vi "AnalyseHeadImpulse2.vi"(0 "head velocity":dbl[](graph), 1 "impulse analysis params":T2={"No. baseline pts"=100, "threshhold"=10.0, "segment length"=300} {"threshhold" format="%.2f"}, 2 "Impulse Analysis Params":T1={"unfiltered vel?"=FALSE, "remove offset? (T)"=FALSE, "analysis method"=enum."polynomial fit", "pre-impulse position"=50, "post-impulse position"=50, "HIT axis"=enum."Pitch", "pre-impulse pts"=50, "post-impulse pts"=50, "polynomial order"=15, "algorithm"=enum."Givens"}, 5 "eye velocity":dbl[](graph), 11 "error in (no error)":errorcluster) -> (3 "impulse analysis params copy":T2={"No. baseline pts"=100, "threshhold"=10.0, "segment length"=9} {"threshhold" format="%.2f"}, 4 "extracted head impulse":dbl[](graph), 6 "extracted eye response":dbl[](graph), 14 "impulse analysis results":T3={"baseline intercept"=3.0, "impulse peak X"=352.0, "len"=400, "+ve ?"=TRUE, "peak velocity"=235.7274415929559} {"peak velocity" format="%.2f"; "impulse peak X" format="%.2f"; "baseline intercept" format="%.2f"}, 15 "error out":errorcluster)   [LabVIEW 2014, in "impulse functions.lvlib"]
uses:
  impulse functions.lvlib
  <vilib>/Analysis/1siggen.llb/Ramp Pattern by Samples.vi
  <vilib>/Analysis/NI_AALPro.lvlib
  <vilib>/Analysis/NI_AALBase.lvlib
panel:
  out "fit segment":dbl[][](graph)
  out "error":i32
  out "mse":dbl format="%.2f"
  out "Polynomial Fit Coefficients":dbl[](array[numeric]) format="%.2f"
  # "Copyright Americo A. Migliaccio (c) 2002 All Rights Reserved by Author"
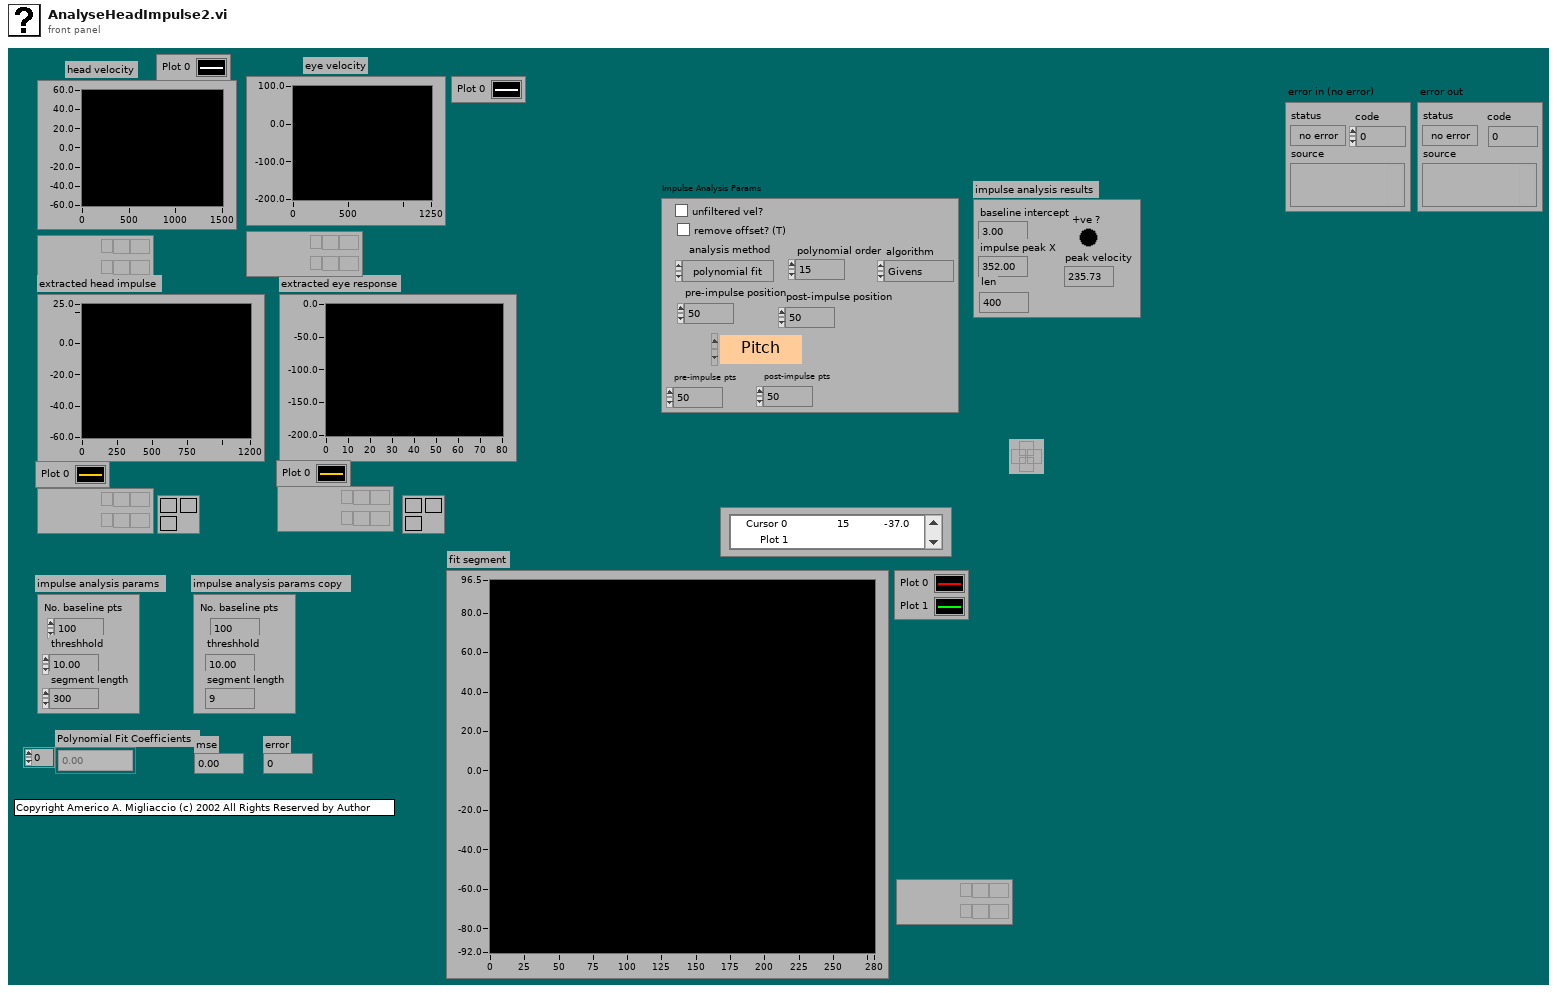
[diagram p1: front panel]
types:
  T1 = cluster{"unfiltered vel?":bool, "remove offset? (T)":bool, "analysis method":enum16{"original", "polynomial fit"}, "pre-impulse position":i32, "post-impulse position":i32, "HIT axis":enum16{"Yaw", "Pitch", "Roll"}, "pre-impulse pts":i32, "post-impulse pts":i32, "polynomial order":i32, "algorithm":enum32{"SVD", "Givens", "Givens2", "Householder", "LU Decomposition", "Cholesky"}}
  T2 = cluster{"No. baseline pts":i32, "threshhold":dbl, "segment length":i32}
  T3 = cluster{"baseline intercept":dbl, "impulse peak X":dbl, "len":i32, "+ve ?":bool, "peak velocity":dbl}
  T4 = enum32{"SVD", "Givens", "Givens2", "Householder", "LU Decomposition", "Cholesky"}
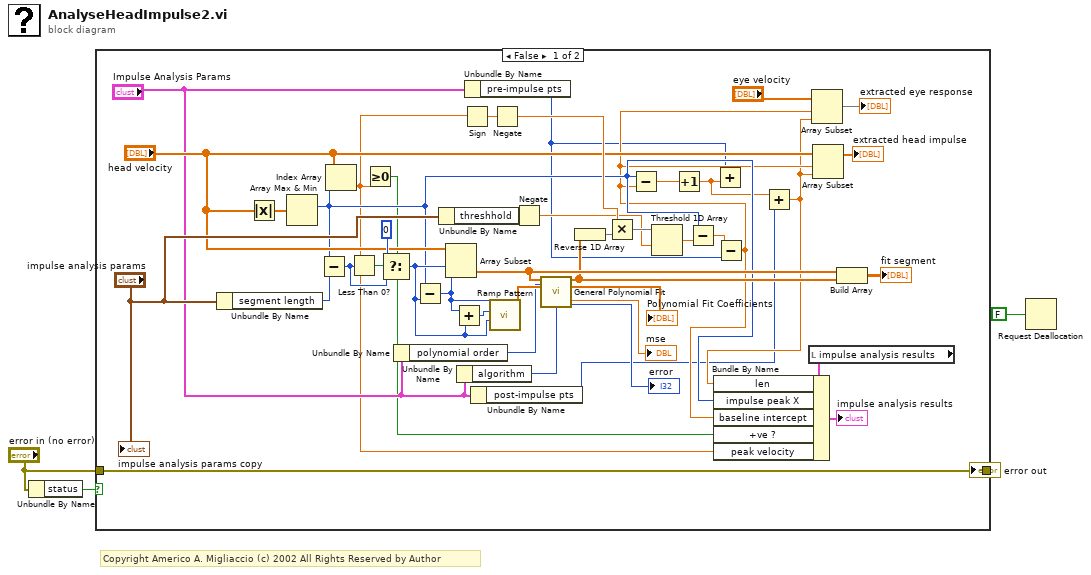
[diagram p0: block diagram]
diagram:
  # "Copyright Americo A. Migliaccio (c) 2002 All Rights Reserved by Author"
  n1 = Unbundle By Name("error in (no error)") -> ("status"=w4:bool)
  n2 = case shown="False" w4 {
    tunnel: "error in (no error)" -> [w40 w48]
    tunnel: [w40 w48] -> w2
    frame False {
      n3 = Unbundle By Name("impulse analysis params") -> ("segment length"=w33:i32)
      n4 = Absolute Value(x="head velocity") -> (abs(x)=w45:dbl[])
      n5 = Array Max & Min(array=w45) -> (max index (indices)=w17:i32)  [unwired: 3 out]
      n6 = Subtract(x=w17, y=w33) -> (x-y=w30:i32)
      n7 = Index Array(array="head velocity", index=w17) -> (element=w5:dbl)
      n8 = Less Than 0?(x=w30) -> (x < 0?=w32:bool)
      n9 = Greater Or Equal To 0?(x=w5) -> (x >= 0?=w6:bool)
      n10 = Select(t=0, s=w32, f=w30) -> (s? t:f=w29:i32)
      n11 = Unbundle By Name("Impulse Analysis Params") -> ("polynomial order"=w9:i32)
      n12 = Subtract(x=w17, y=w29) -> (x-y=w19:i32)
      n13 = Unbundle By Name("impulse analysis params") -> ("threshhold"=w27:dbl)
      n14 = Array Subset(array="head velocity", index=w29, length=w19) -> (w34:dbl[])
      n15 = Add(x=w19, y=w29) -> (x+y=w41:i32)
      n16 = Unbundle By Name("Impulse Analysis Params") -> ("algorithm"=w8:T4)
      n17 = Sign(1:w5) -> (0:w23:dbl)
      n18 = Unbundle By Name("Impulse Analysis Params") -> ("pre-impulse pts"=w11:i32)
      n19 = Unbundle By Name("Impulse Analysis Params") -> ("post-impulse pts"=w10:i32)
      n20 = call-poly <vilib>:"Ramp Pattern.vi"("start"=w29, "end"=w41, "samples"=w19) -> ("Ramp Pattern"=w39:dbl[])  [unwired: 7 in, 1 out]
      n21 = Negate(x=w23) -> (-x=w22:dbl)
      n22 = Negate(x=w27) -> (-x=w21:dbl)
      n23 = call <vilib>:"General Polynomial Fit.vi"("Y"=w34, "polynomial order"=w9, "X"=w39, "algorithm"=w8) -> ("Best Polynomial Fit"=w28:dbl[], "Polynomial Coefficients"=→"Polynomial Fit Coefficients":dbl[], "residue"=→"mse":dbl, "error"=→"error":i32)  [unwired: 8 in]
      n24 = Reverse 1D Array(array=w28) -> (reversed array=w25:dbl[])
      n25 = Multiply(x=w22, y=w25) -> (x*y=w24:dbl[])
      n26 = Threshold 1D Array(2:w21, 3:w24) -> (0:w18:dbl)  [unwired: 1 in]
      n27 = Subtract(x=w17, y=w18) -> (x-y=w15:dbl)
      n28 = Subtract(x=w15, y=w11) -> (x-y=w14:dbl)
      n29 = Subtract(x=w17, y=w14) -> (x-y=w16:dbl)
      n30 = Increment(x=w16) -> (x+1=w13:dbl)
      n31 = Add(x=w11, y=w13) -> ()  [unwired: 1 out]
      n32 = Add(x=w13, y=w10) -> (x+y=w12:dbl)
      n33 = local read "impulse analysis results"() -> (w44:T3)
      n34 = Bundle By Name(cluster=w44, "len"=w12, "impulse peak X"=w17, "baseline intercept"=w14, "+ve ?"=w6, "peak velocity"=w5) -> (→"impulse analysis results":T3)
      n35 = Array Subset(array="eye velocity", index=w14, length=w12) -> (→"extracted eye response":dbl[])
      n36 = Array Subset(array="head velocity", index=w14, length=w12) -> (→"extracted head impulse":dbl[])
      n37 = Build Array(w34, w28) -> (→"fit segment":dbl[][])
      "impulse analysis params copy" <- "impulse analysis params"
    }
    frame True {
    }
  }
  "error out" <- w2
  n38 = Request Deallocation(FALSE ("flag")) -> ()
